vi "Test TLS.vi"() -> ()   [LabVIEW 2020]
panel:
  out "remote port":u16
  out "error out":errorcluster
  out "Headers":string
  out "client certificate chain":cluster{"certificate":u8[]}[](array[cluster])
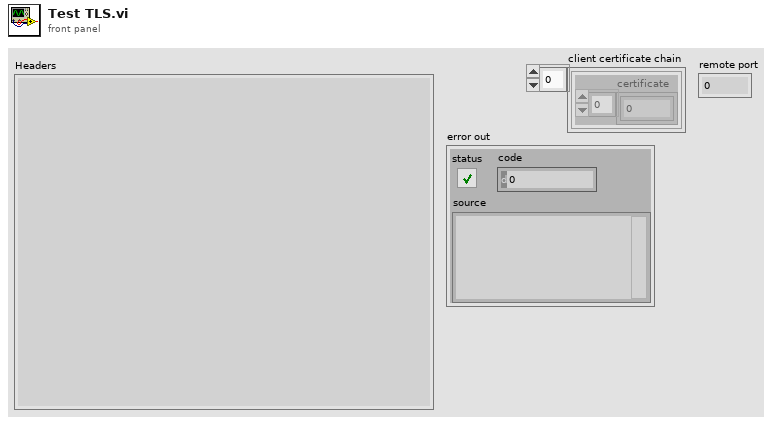
[diagram p1: front panel]
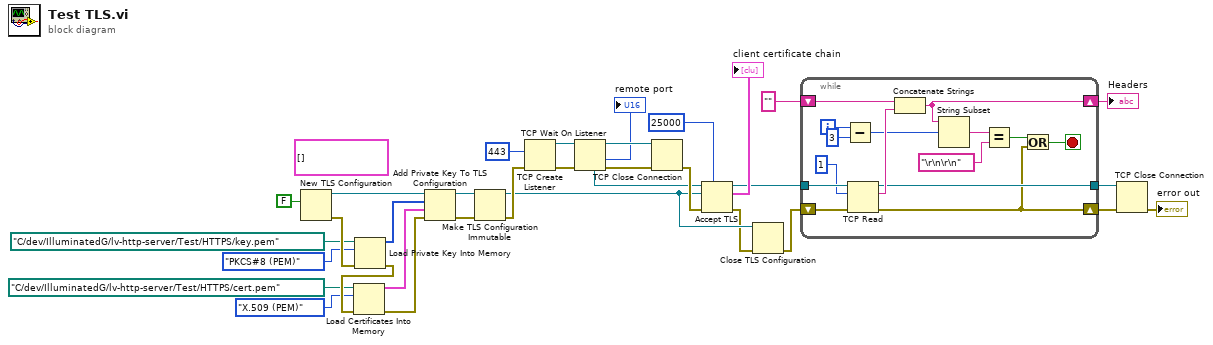
[diagram p0: block diagram]
diagram:
  (unwired) cluster{"certificate":u8[]}[] [] ("certificate chain")
  n1 = New TLS Configuration(10:FALSE ("load OS trusted CAs?")) -> (0:w33:errorcluster, 3:w27:refnum<k36>)  [unwired: 1 in]
  n2 = Load Private Key Into Memory(8:w33, 10:enum32{"PKCS#8 (PEM)", "PKCS#8 (DER)"}."PKCS#8 (PEM)" ("format"), 11:path "C:/dev/IlluminatedG/lv-http-server/Test/HTTPS/key.pem" ("path")) -> (0:w32:errorcluster, 3:w26:u8[])  [unwired: 1 in]
  n3 = Load Certificates Into Memory(8:w32, 10:enum32{"X.509 (PEM)"}."X.509 (PEM)" ("format"), 11:path "C:/dev/IlluminatedG/lv-http-server/Test/HTTPS/cert.pem" ("path")) -> (0:w22:errorcluster, 3:w2:cluster{"certificate":u8[]}[])
  n4 = Add Private Key To TLS Configuration(8:w22, 9:w2, 10:w26, 11:w27) -> (0:w21:errorcluster, 3:w23:refnum<k36>)
  n5 = Make TLS Configuration Immutable(8:w21, 11:w23) -> (0:w20:errorcluster, 3:w11:refnum<k36>)
  n6 = TCP Create Listener(8:w20, 10:u16 443 ("port")) -> (0:w19:errorcluster, 3:w30:refnum<k5>)  [unwired: 3 in, 1 out]
  n7 = TCP Wait On Listener(8:w19, 11:w30) -> (0:w17:errorcluster, 1:→"remote port":u16, 3:w18:refnum<k5>, 4:w15:refnum<k5>)  [unwired: 2 in, 1 out]
  n8 = TCP Close Connection(connection ID=w18, error in (no error)=w17) -> (error out=w16:errorcluster)  [unwired: 1 in, 1 out]
  n9 = Accept TLS(7:25000 ("timeout ms"), 8:w16, 10:w11, 11:w15) -> (0:w10:errorcluster, 2:→"client certificate chain":cluster{"certificate":u8[]}[], 3:w13:refnum<k5>)
  n10 = Close TLS Configuration(8:w10, 11:w11) -> (0:w9:errorcluster)
  n11 = while {
    tunnel: w13 -> [w48]
    shift-right: [w34] -> w6
    shift-left: w9 -> [w47]
    shift-right: [w41] -> w8
    shift-left: "" -> [w44]
    tunnel: [w36] -> w7
    i -> [w43]
    stop <- w35 stop-if-true
    n12 = Subtract(x=w43, y=3) -> (x-y=w40:i32)
    n13 = TCP Read(connection ID=w48, bytes to read=1, error in (no error)=w47) -> (connection ID out=w36:refnum<k5>, data out=w45:string, error out=w34:errorcluster)  [unwired: 2 in]
    n14 = Concatenate Strings(w44, w45) -> (w41:string)
    n15 = String Subset(string=w41, offset (0)=w40) -> (substring=w38:string)  [unwired: 1 in]
    n16 = Equal?(x=w38, y="\r\n\r\n") -> (x = y?=w37:bool)
    n17 = Or(x=w37, y=w34) -> (x .or. y?=w35:bool)
  }
  "Headers" <- w8
  n18 = TCP Close Connection(connection ID=w7, error in (no error)=w6) -> (error out=→"error out":errorcluster)  [unwired: 1 in, 1 out]
